vi "PH_SSAC.Back Ground.vi"(0 "i ref in":refnum<vi>, 5 "error in":errorcluster) -> (14 "i ref out":refnum<vi>, 19 "error out":errorcluster)   [LabVIEW 2014, in "PH_SSAC.lvlib"]
doc: "This VI calculates background stuff."
uses:
  PH_SSAC.lvlib
  PH_SSAC.Background Data.ctl
  PH_Basics/PH_Common/PH_Common.lvlib
panel:
  in  "Background Calibration Data":T1={"Date"="", "Time"="", "Frame Main"={"x"=0, "dx"=0, "y"=0, "dy"=0}, "dt [fs]"=0.0, "Calibration Factor [fs/pixel]"=0.0, "Signal"=array[1280 elements], "Frame Background"={"x"=0, "dx"=100, "y"=400, "dy"=250}}
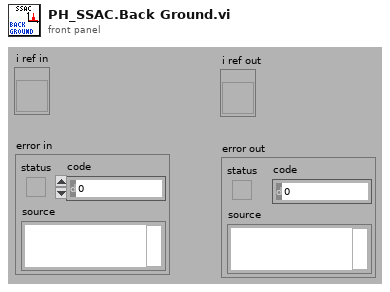
[diagram p1: front panel]
types:
  T1 = typedef "PH_SSAC.lvlib/PH_SSAC.Background Data.ctl" = cluster{"Date":string, "Time":string, "Frame Main":cluster{"x":u32, "dx":u32, "y":u32, "dy":u32}, "dt [fs]":dbl, "Calibration Factor [fs/pixel]":dbl, "Signal":dbl[], "Frame Background":cluster{"x":u32, "dx":u32, "y":u32, "dy":u32}}
  T2 = typedef "PH_SSAC.lvlib/PH_SSAC.i attribute.ctl" = cluster{"GUI Refs":cluster{"Delete":refnum<vi>, "Global On":refnum<vi>, "Cam Source":refnum<vi>, "Frame Main Signal":refnum<vi>, "Frame Background":refnum<vi>, "dt (Gauss smooth)":refnum<vi>, "Calibration Factor":refnum<vi>, "Background acquire":refnum<vi>, "Threshold":refnum<vi>, "Time evolution of mean pulse duration":refnum<vi>, "Mean Pulse Duration":refnum<vi>, "Main signal":refnum<vi>, "Current Pulse Duration":refnum<vi>, "Processed":refnum<vi>, "Saturation":refnum<vi>, "# for Average":refnum<vi>, "Position":refnum<vi>, "BG Status":refnum<vi>, "Save BG data":refnum<vi>, "Read BG Data":refnum<vi>, "Background Calibration Data":refnum<vi>}, "Images":cluster{"OP Image":T3, "GUI Image":T3, "PSDB Image":T3}, "Global On?":bool, "Frame Main":cluster{"x":u32, "dx":u32, "y":u32, "dy":u32}, "Frame Background":cluster{"x":u32, "dx":u32, "y":u32, "dy":u32}, "dt [fs]":dbl, "Calibration Factor [fs/pixel]":dbl, "Threshold":dbl, "Time evolution of mean pulse duration [fs]":dbl[], "Main Signal":cluster{"Time for Main":dbl[], "Signal":dbl[]}, "Processed":bool, "Current Pulse Duration [fs]":dbl, "# for Average":i32, "Position":i32, "Pulse Durations [fs]":dbl[], "BG":cluster{"Acquire?":bool, "Background Calibration Data":T1, "Save Data":bool}}
  T3 = typedef "IMAQ Image.ctl" = refnum<image>
  T4 = enum16{"open", "replace", "create", "open or create", "replace or create", "replace or create with confirmation"}
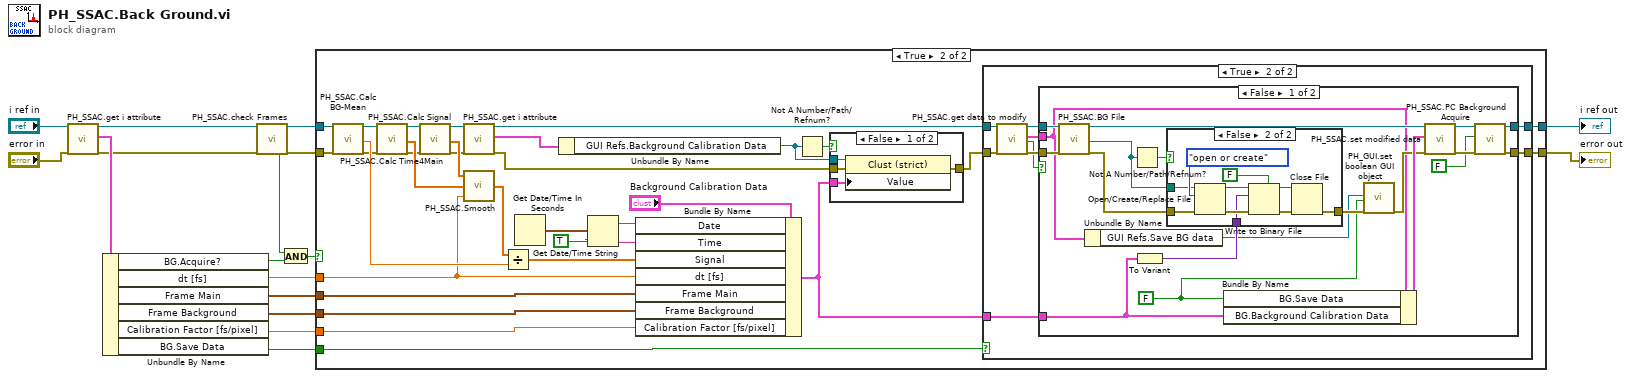
[diagram p0: block diagram]
diagram:
  n1 = call "PH_SSAC.get i attribute.vi"("i ref in"="i ref in", "error in (no error)"="error in") -> ("i ref out"=w8:refnum<vi>, "i attribute"=w15:T2, "error out"=w9:errorcluster)  [unwired: 15 in]
  n2 = Unbundle By Name(w15) -> ("BG.Acquire?"=w4:bool, "dt [fs]"=w12:dbl, "Frame Main"=w10:cluster{"x":u32, "dx":u32, "y":u32, "dy":u32}, "Frame Background"=w1:cluster{"x":u32, "dx":u32, "y":u32, "dy":u32}, "Calibration Factor [fs/pixel]"=w11:dbl, "BG.Save Data"=w7:bool)
  n3 = call "PH_SSAC.check Frames.vi"("i ref in"=w8, "error in"=w9) -> ("All ok?"=w3:bool, "i ref out"=w5:refnum<vi>, "error out"=w6:errorcluster)  [unwired: 11 in, 4 out]
  n4 = And(x=w3, y=w4) -> (x .and. y?=w2:bool)
  n5 = case shown="True" w2 {
    tunnel: [w18 w32] -> w14
    tunnel: [w19 w31] -> w13
    tunnel: w6 -> [w18 w43]
    tunnel: w5 -> [w19 w42]
    tunnel: w12 -> [_ w35]
    tunnel: w10 -> [_ w36]
    tunnel: w11 -> [_ w34]
    tunnel: w7 -> [_ w26]
    tunnel: w1 -> [_ w20]
    frame False {
    }
    frame True {
      n6 = call "PH_SSAC.Calc BG-Mean.vi"("i ref in"=w42, "error out"=w43) -> ("i ref out"=w46:refnum<vi>, "BG Mean Value [Pixel]"=w51:dbl, "error out"=w47:errorcluster)  [unwired: 15 in]
      n7 = call "PH_SSAC.Calc Time4Main.vi"("i ref in"=w46, "error in"=w47) -> ("i ref out"=w45:refnum<vi>, "Time for Main [fs]"=w48:dbl[], "error out"=w44:errorcluster)  [unwired: 15 in]
      n8 = call "PH_SSAC.Calc Signal.vi"("i ref in"=w45, "error in"=w44) -> ("i ref out"=w30:refnum<vi>, "Main Frame Linear Averages [pixel]"=w49:dbl[], "error out"=w28:errorcluster)  [unwired: 15 in]
      n9 = call "PH_SSAC.get i attribute.vi"("i ref in"=w30, "error in (no error)"=w28) -> ("i ref out"=w29:refnum<vi>, "i attribute"=w25:T2, "error out"=w27:errorcluster)  [unwired: 15 in]
      n10 = call "PH_SSAC.Smooth.vi"("dt [fs]"=w35, "Time [fs]"=w48, "Frame Linear Averages [pixel]"=w49) -> ("Signal*Smooth"=w50:dbl[])
      n11 = Divide(x=w50, y=w51) -> (x/y=w33:dbl[])
      n12 = Get Date/Time In Seconds() -> (seconds since 1Jan1904=w41:timestamp)
      n13 = Unbundle By Name(w25) -> ("GUI Refs.Background Calibration Data"=w21:refnum<vi>)
      n14 = Get Date/Time String(seconds (now)=w41, want seconds? (F)=TRUE) -> (date string=w38:string, time string=w37:string)  [unwired: 1 in]
      n15 = Bundle By Name(cluster="Background Calibration Data", "Date"=w38, "Time"=w37, "Signal"=w33, "dt [fs]"=w35, "Frame Main"=w36, "Frame Background"=w20, "Calibration Factor [fs/pixel]"=w34) -> (w23:T1)
      n16 = Not A Number/Path/Refnum?(number/path/refnum=w21) -> (NaN/Path/Refnum?=w22:bool)
      n17 = case shown="False" w22 {
        tunnel: w27 -> [w55 w56]
        tunnel: [w54 w56] -> w24
        tunnel: w21 -> [w53 _]
        tunnel: w23 -> [w52 _]
        frame False {
          n18 = property class="Clust (strict)"(reference=w53, error in=w55, "Value"=w52) -> (error out=w54:errorcluster)  [unwired: 1 out]
        }
        frame True {
        }
      }
      n19 = case shown="True" w26 {
        tunnel: w23 -> [_ w67]
        tunnel: [w57 w64] -> w32
        tunnel: [w58 w63] -> w31
        tunnel: w29 -> [w58 w60]
        tunnel: w24 -> [w57 w59]
        frame False {
        }
        frame True {
          n20 = call "PH_SSAC.get data to modify.vi"("i ref in"=w60, "error in (no error)"=w59) -> ("i ref out"=w65:refnum<vi>, "i attribute"=w61:T2, "timed out"=w62:bool, "error out"=w66:errorcluster)  [unwired: 14 in]
          n21 = case shown="False" w62 {
            tunnel: w67 -> [w79 _]
            tunnel: w66 -> [w83 w98]
            tunnel: w65 -> [w82 w99]
            tunnel: [w75 w98] -> w64
            tunnel: [w76 w99] -> w63
            tunnel: w61 -> [w72 _]
            frame False {
              w70 = FALSE ("BG.Save Data")
              n22 = call "PH_SSAC.BG File.vi"("i ref in"=w82, "error in"=w83) -> ("i ref out"=w81:refnum<vi>, "BG File"=w68:path, "error out"=w85:errorcluster)  [unwired: 15 in]
              n23 = Unbundle By Name(w72) -> ("GUI Refs.Save BG data"=w71:refnum<vi>)
              n24 = Not A Number/Path/Refnum?(number/path/refnum=w68) -> (NaN/Path/Refnum?=w69:bool)
              n25 = To Variant(anything=w79) -> (Variant=w86:variant)
              n26 = case shown="False" w69 {
                tunnel: w86 -> [_ w93]
                tunnel: w85 -> [w87 w91]
                tunnel: [w87 w90] -> w84
                tunnel: w68 -> [_ w88]
                frame True {
                }
                frame False {
                  n27 = Open/Create/Replace File(file path (use dialog)=w88, error in=w91, operation (0:open)=T4."open or create") -> (refnum out=w97:refnum<file>, error out=w96:errorcluster)  [unwired: 3 in, 1 out]
                  n28 = Write to Binary File(file (use dialog)=w97, data=w93, error in=w96, 5:FALSE ("prepend array or string size? (T)")) -> (refnum out=w94:refnum<file>, error out=w95:errorcluster)  [unwired: 2 in, 1 out]
                  n29 = Close File(refnum=w94, error in=w95) -> (error out=w90:errorcluster)  [unwired: 1 out]
                }
              }
              n30 = Bundle By Name(cluster=w72, "BG.Save Data"=w70, "BG.Background Calibration Data"=w79) -> (w80:T2)
              n31 = call "PH_GUI.set boolean GUI object.vi"("Boolean Knob GUI Ref"=w71, "Value"=w70, "error in (no error)"=w84) -> ("error out"=w73:errorcluster)  [unwired: 16 in]
              n32 = call "PH_SSAC.set modified data.vi"("i ref in"=w81, "i attribute"=w80, "error in (no error)"=w73) -> ("i ref out"=w77:refnum<vi>, "error out"=w78:errorcluster)  [unwired: 15 in]
              n33 = call "PH_SSAC.PC Background Acquire.vi"("i ref in"=w77, "BG Acquire"=FALSE, "error IO"=w78) -> ("i ref out"=w76:refnum<vi>, "error out"=w75:errorcluster)  [unwired: 15 in]
            }
            frame True {
            }
          }
        }
      }
    }
  }
  "error out" <- w14
  "i ref out" <- w13
